vi "实验6.1.vi"() -> ()   [LabVIEW 2017]
panel:
  out "倒计时":timestamp format="%<%M:%S>T"
  in  "停止":bool
  out "布尔":bool
  in  "开始倒计时":bool
  in  "定时时间选择":enum16{"20秒", "10秒", "6秒"}(ring)
  # "倒计时器"
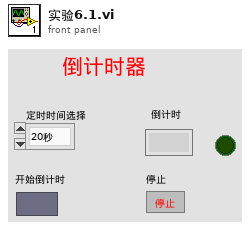
[diagram p1: front panel]
types:
  T1 = enum8{"Enabled", "Disabled", "Disabled and Grayed Out"}
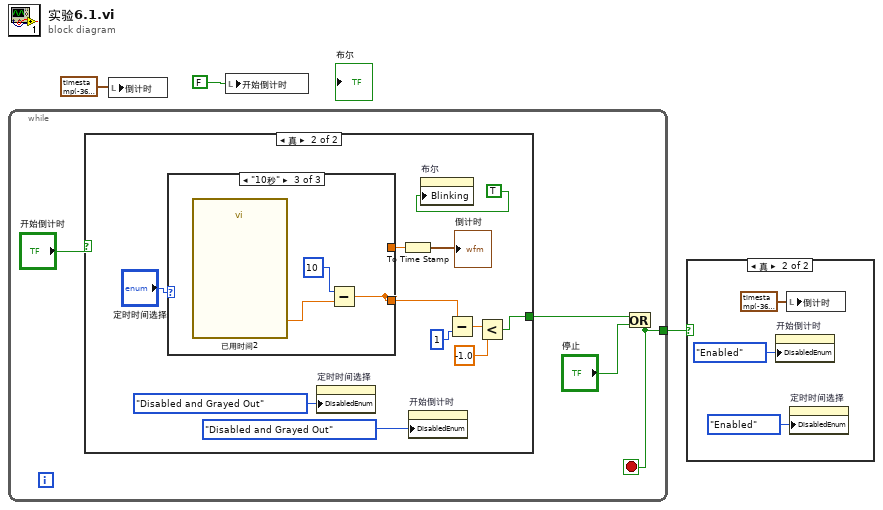
[diagram p0: block diagram]
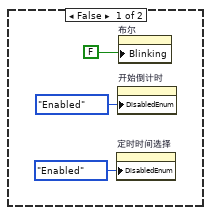
[diagram p3: hidden frame]
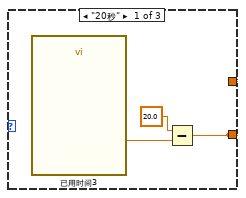
[diagram p4: hidden frame]
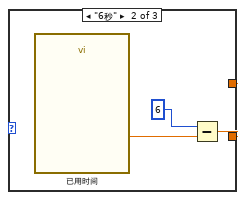
[diagram p5: hidden frame]
diagram:
  n1 = while {
    tunnel: [w5] -> w2
    stop <- w5 stop-if-true
    n2 = case shown="真" "开始倒计时" {
      tunnel: [_ w13] -> w4
      frame False {
        n3 = property on="定时时间选择" class="Enum (严格)"("DisabledEnum"=T1."Enabled" ("禁用")) -> ()  [unwired: 2 in, 2 out]
        n4 = property on="开始倒计时" class="Bool (严格)"("DisabledEnum"=T1."Enabled" ("禁用")) -> ()  [unwired: 2 in, 2 out]
        n5 = property on="布尔" class="Bool (严格)"("Blinking"=FALSE) -> ()  [unwired: 2 in, 2 out]
      }
      frame True {
        n6 = case shown="\"10秒\"" "定时时间选择" {
          tunnel: [w22 w25 w28] -> w17
          tunnel: [w22 w25 w28] -> w12
          frame "20秒" {
            n7 = call "已用时间3"() -> ("Elapsed Time (s)"=w24:dbl)  [unwired: 12 in, 7 out]
            n8 = Subtract(x=20.0, y=w24) -> (x-y=w22:dbl)
          }
          frame "6秒" {
            n9 = call "已用时间"() -> ("Elapsed Time (s)"=w27:dbl)  [unwired: 12 in, 7 out]
            n10 = Subtract(x=6, y=w27) -> (x-y=w25:dbl)
          }
          frame "10秒" {
            n11 = call "已用时间2"() -> ("Elapsed Time (s)"=w30:dbl)  [unwired: 12 in, 7 out]
            n12 = Subtract(x=10, y=w30) -> (x-y=w28:dbl)
          }
        }
        n13 = property on="定时时间选择" class="Enum (严格)"("DisabledEnum"=T1."Disabled and Grayed Out" ("禁用")) -> ()  [unwired: 2 in, 2 out]
        n14 = To Time Stamp(1:w12) -> (0:→"倒计时":timestamp)
        n15 = property on="开始倒计时" class="Bool (严格)"("DisabledEnum"=T1."Disabled and Grayed Out" ("禁用")) -> ()  [unwired: 2 in, 2 out]
        n16 = property on="布尔" class="Bool (严格)"("Blinking"=TRUE) -> ()  [unwired: 2 in, 2 out]
        n17 = Subtract(x=w17, y=1) -> (x-y=w15:dbl)
        n18 = Less?(x=w15, y=-1.0) -> (x < y?=w13:bool)
      }
    }
    n19 = Or(x=w4, y="停止") -> (x .or. y?=w5:bool)
  }
  n20 = local write "倒计时"(timestamp(-3599.000343322754 s since 1904-01-01) ("倒计时")) -> ()
  n21 = local write "开始倒计时"(FALSE ("开始倒计时")) -> ()
  n22 = case shown="真" w2 {
    frame False {
    }
    frame True {
      n23 = property on="开始倒计时" class="Bool (严格)"("DisabledEnum"=T1."Enabled" ("禁用")) -> ()  [unwired: 2 in, 2 out]
      n24 = local write "倒计时"(timestamp(-3599.0002608299255 s since 1904-01-01) ("倒计时")) -> ()
      n25 = property on="定时时间选择" class="Enum (严格)"("DisabledEnum"=T1."Enabled" ("禁用")) -> ()  [unwired: 2 in, 2 out]
    }
  }
